vi "Status.vi"(8 "error in (no error)":errorcluster, 10 "Internal?":bool, 11 "Lauda Settings":T1) -> (0 "error out":errorcluster, 1 "Connection Error":bool, 2 "Running":bool, 3 "Lauda Settings":T1, 4 "Temp":dbl, 5 "No external Sensor":bool, 6 "Pump Speed":i32)   [LabVIEW 2021, in "Lauda TCU.lvlib"]
uses:
  Lauda TCU.lvlib
  Lauda Settings.ctl
  <vilib>/Utility/error.llb/DialogType.ctl
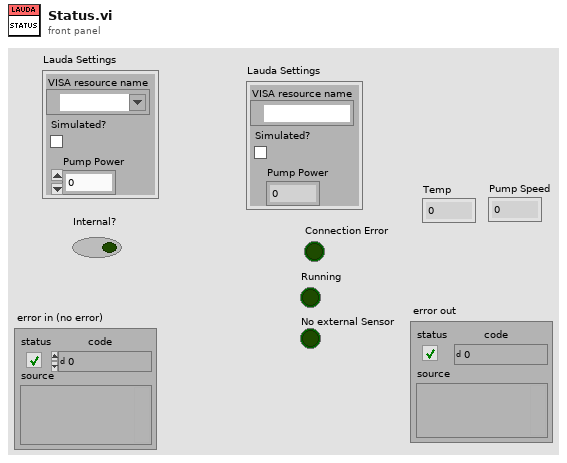
[diagram p1: front panel]
types:
  T1 = typedef "Lauda TCU.lvlib/Lauda Settings.ctl" = cluster{"VISA resource name":refnum<visa-resource-name>, "Simulated?":bool, "Pump Power":i32}
  T2 = typedef "DialogType.ctl" = u16
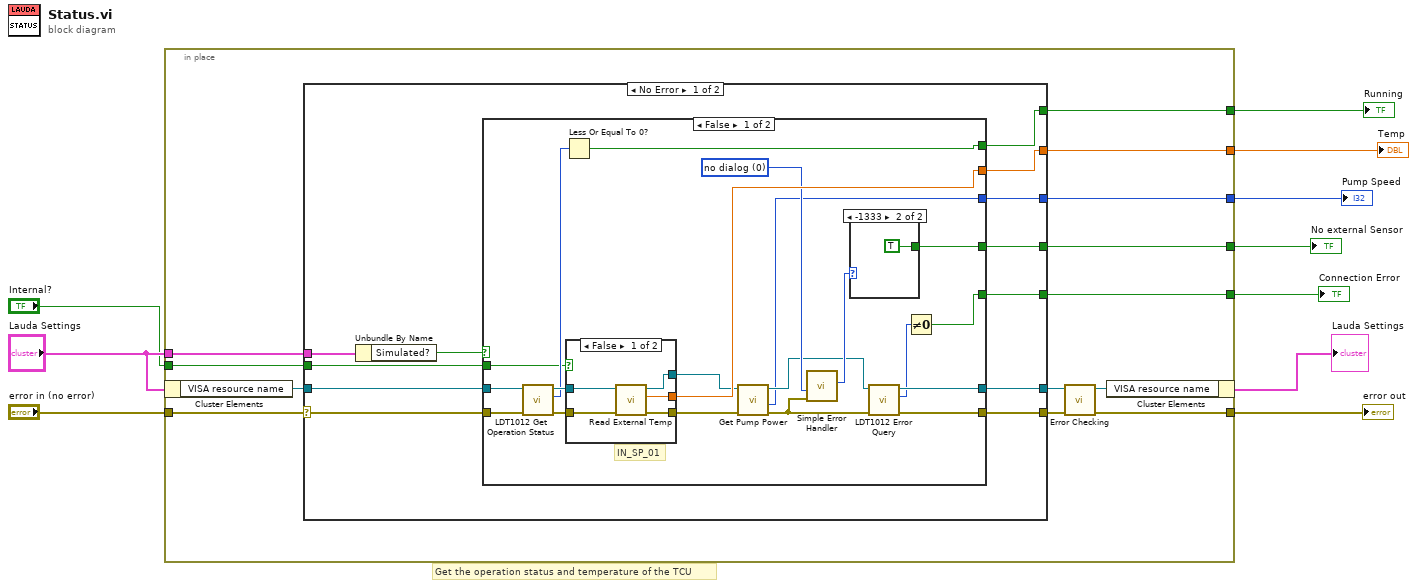
[diagram p0: block diagram]
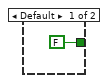
[diagram p2: hidden frame]
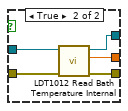
[diagram p3: hidden frame]
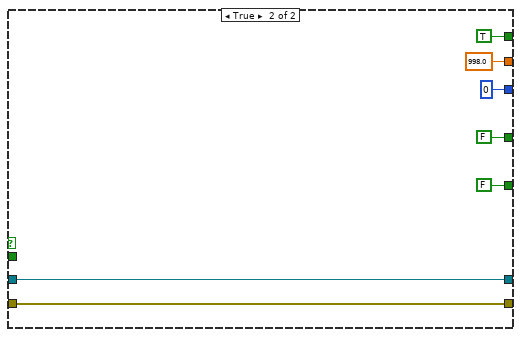
[diagram p4: hidden frame]
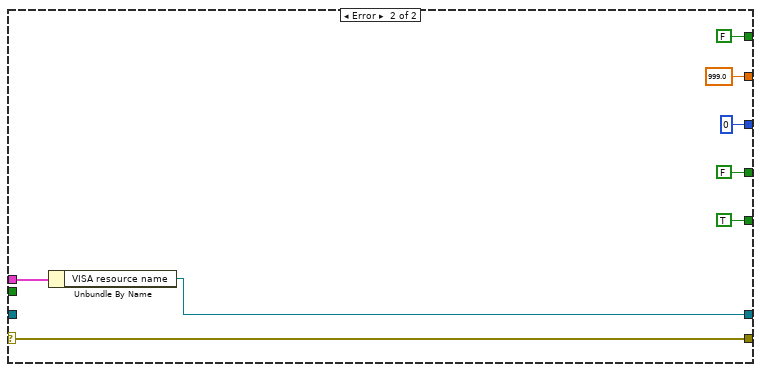
[diagram p5: hidden frame]
diagram:
  # "Get the operation status and temperature of the TCU"
  n1 = in-place {
    in-place-border: "error in (no error)" -> [w23]
    in-place-border: [w20] -> w9
    in-place-border: "Lauda Settings" -> [w19]
    in-place-border: [w18] -> w8
    in-place-border: [w17] -> w7
    in-place-border: [w16] -> w6
    in-place-border: [w15] -> w5
    in-place-border: [w14] -> w4
    in-place-border: "Internal?" -> [w11]
    n2 = in-place-cluster #1("Lauda Settings") -> ("VISA resource name"=w13:refnum<visa-resource-name>)
    n3 = case shown="No Error" w23 {
      selector: w23 -> [w35 w82]
      tunnel: w19 -> [w33 w81]
      tunnel: [w34 w82] -> w21
      tunnel: [w32 w80] -> w22
      tunnel: [w30 TRUE] -> w18
      tunnel: [w29 FALSE] -> w17
      tunnel: [w28 999.0 ("Internal Bath Temperature")] -> w16
      tunnel: [w27 FALSE] -> w15
      tunnel: [w26 0 ("Pump Speed")] -> w14
      tunnel: w13 -> [w25 _]
      tunnel: w11 -> [w24 _]
      frame No Error {
        n4 = Unbundle By Name(w33) -> ("Simulated?"=w31:bool)
        n5 = case shown="False" w31 {
          tunnel: w35 -> [w54 w74]
          tunnel: [w50 w74] -> w34
          tunnel: [w51 w73] -> w32
          tunnel: w25 -> [w55 w73]
          tunnel: [w48 FALSE] -> w30
          tunnel: [w38 TRUE] -> w29
          tunnel: [w47 998.0 ("Internal Bath Temperature")] -> w28
          tunnel: [w45 FALSE] -> w27
          tunnel: [w39 0 ("Pump Speed")] -> w26
          tunnel: w24 -> [w36 _]
          frame False {
            w44 = T2 0 items=["no dialog", "OK message", "continue or stop message", "OK message + warnings", "continue/stop + warnings"] ("type of dialog (OK msg:1)")
            # "IN_SP_01"
            n6 = call "LDT1012 Get Operation Status.vi"("error in (no error)"=w54, "VISA session"=w55) -> ("error out"=w52:errorcluster, "Get Operation Status"=w37:u8, "dup VISA session"=w53:refnum<visa-resource-name>)  [unwired: 7 in]
            n7 = Less Or Equal To 0?(x=w37) -> (x <= 0?=w38:bool)
            n8 = case shown="False" w36 {
              tunnel: w53 -> [w61 w67]
              tunnel: w52 -> [w60 w66]
              tunnel: [w62 w65] -> w43
              tunnel: [w59 w64] -> w41
              tunnel: [w58 w63] -> w47
              frame False {
                n9 = call "Read External Temp.vi"("error in (no error)"=w60, "VISA session"=w61) -> ("error out"=w59:errorcluster, "External PT100 Temperature"=w58:dbl, "dup VISA session"=w62:refnum<visa-resource-name>)  [unwired: 7 in]
              }
              frame True {
                n10 = call "LDT1012 Read Bath Temperature Internal.vi"("error in (no error)"=w66, "VISA session"=w67) -> ("error out"=w64:errorcluster, "Internal Bath Temperature"=w63:dbl, "dup VISA session"=w65:refnum<visa-resource-name>)  [unwired: 7 in]
              }
            }
            n11 = call "Get Pump Power.vi"("error in (no error)"=w41, "VISA session"=w43) -> ("error out"=w40:errorcluster, "Pump Speed"=w39:i32, "dup VISA session"=w42:refnum<visa-resource-name>)  [unwired: 6 in, 1 out]
            n12 = call <vilib>:"Simple Error Handler.vi"("type of dialog (OK msg:1)"=w44, "error in (no error)"=w40) -> ("code out"=w46:i32)  [unwired: 3 in, 4 out]
            n13 = case shown="-1333" w46 {
              tunnel: [FALSE TRUE] -> w45
              frame Default {
              }
              frame -1333 {
              }
            }
            n14 = call "LDT1012 Error Query.vi"("error in (no error)"=w40, "VISA session"=w42) -> ("error out"=w50:errorcluster, "Error"=w49:u8, "dup VISA session"=w51:refnum<visa-resource-name>)  [unwired: 5 in, 2 out]
            n15 = Not Equal To 0?(x=w49) -> (x != 0?=w48:bool)
          }
          frame True {
          }
        }
      }
      frame Error {
        n16 = Unbundle By Name(w81) -> ("VISA resource name"=w80:refnum<visa-resource-name>)
      }
    }
    n17 = call "Error Checking.vi"("error in (no error)"=w21, "VISA resource name"=w22) -> ("error out"=w20:errorcluster, "VISA resource name"=w12:refnum<visa-resource-name>)  [unwired: 7 in, 1 out]
    n18 = in-place-cluster #1("VISA resource name"=w12) -> (→"Lauda Settings":T1)
  }
  "error out" <- w9
  "Connection Error" <- w8
  "Running" <- w7
  "Temp" <- w6
  "No external Sensor" <- w5
  "Pump Speed" <- w4
